vi "Auto Drive.vi"(6 "2nd Gear?":dbl, 7 "Async?":dbl, 8 "X Speed":dbl, 9 "Y Speed":dbl, 10 "Heading Target":dbl, 11 "Distance Target":dbl) -> (3 "Finished?":bool)   [LabVIEW 2017]
uses:
  Common Code/Drivetrain Mode.ctl
  Robot Global Data.vi
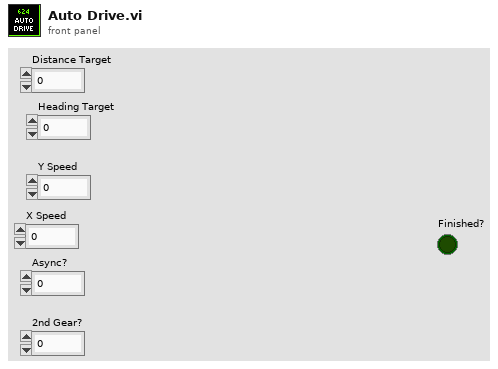
[diagram p1: front panel]
types:
  T1 = typedef "Drivetrain Mode.ctl" = enum16{"Manual", "Gyro Steer", "PID Drive", "Distance Drive", "Autonomous"}
  T2 = typedef "Dashboard Status Data.ctl" = cluster{"Elevator Status Cluster":T3, "Drivetrain Status Cluster":T6, "Intake Status Cluster":T8, "Climb Status Cluster":T11, "Intake PDP Info":T12}
  T3 = typedef "Elevator Status Cluster.ctl" = cluster{"Finished":bool, "Elevator Power":dbl, "Elevator State":T4, "Elevator Mode":T5, "Elevator Height":dbl, "At Bottom?":bool, "At Top?":bool, "Scale high?":bool, "PID Output":dbl}
  T4 = typedef "Elevator State.ctl" = enum16{"Idle", "Ground", "Mid", "Scale", "Switch"}
  T5 = typedef "Elevator Mode.ctl" = enum16{"Semi Auto", "Manual", "Auto"}
  T6 = typedef "Drivetrain Status Cluster.ctl" = cluster{"Throttle (Y)":dbl, "Steer (X)":dbl, "Drivetrain Mode":T1, "Brake?":bool, "Distance Drive Complete?":bool, "PID Drive Complete?":bool, "Creep Mode?":bool, "Gyro Steer Complete?":bool, "Gyro":dbl, "X Max Output":dbl, "X Min Output":dbl, "Y Max Output ":dbl, "Y Min Output":dbl, "Heading Target":dbl, "Distance Target":dbl, "2nd Gear":bool, "Drivetrain Encoder Values":T7}
  T7 = typedef "DT Encoder Values.ctl" = cluster{"Left Encoder":cluster{"Distance":dbl, "Speed":dbl, "Tick":dbl}, "Right Encoder":cluster{"Distance":dbl, "Speed":dbl, "Tick":dbl}}
  T8 = typedef "Intake Status Cluster.ctl" = cluster{"Intake Mode":T9, "Intake States":T10, "Intake Current Angle":dbl, "Cube In Posession?":bool, "Intake Wrist Up?":bool}
  T9 = typedef "Intake Mode.ctl" = enum16{"Auto", "Semi Auto", "Manual"}
  T10 = typedef "Intake States.ctl" = enum16{"Zero", "Override Angle", "Idle", "Drop Mid", "Drop Low", "Outtake", "Intake"}
  T11 = typedef "Climb Status Cluster.ctl" = cluster{"Climb":bool, "Time Remaining":dbl, "Button Pressed":bool}
  T12 = typedef "Intake PDP Info.ctl" = cluster{"Voltage Percent Output":dbl, "Output Voltage":dbl, "Bus Voltage":dbl, "Device ID":dbl, "Output Current":dbl, "Sensor Velocity":dbl, "Sensor Position":dbl, "Pulse Width Position":dbl, "Pulse Width Velocity":dbl, "Temperature":dbl, "Inverted?":bool}
  T13 = typedef "Drivetrain Command Cluster.ctl" = cluster{"Y Power":dbl, "Turn Power":dbl, "Drivetrain Mode":T1, "2nd Gear":bool, "Y Min Output":dbl, "Y Max Output":dbl, "X Min Output":dbl, "X Max Output":dbl, "Heading Target":dbl, "Distance Target":dbl, "Brake?":bool, "Zero Gyro":bool}
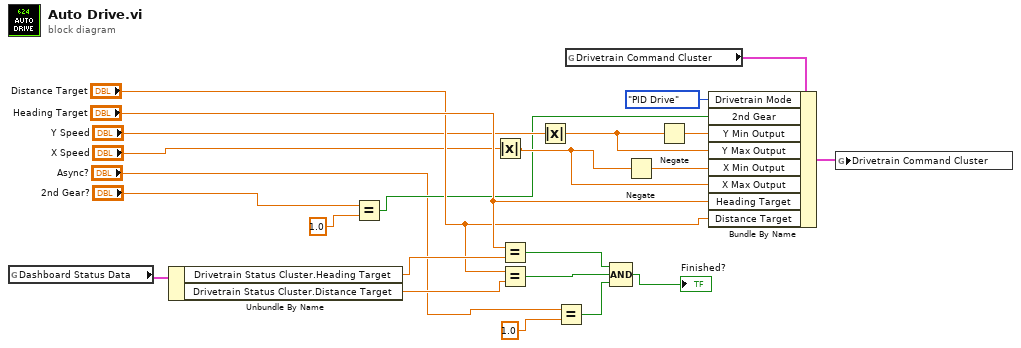
[diagram p0: block diagram]
diagram:
  n1 = global read "Robot Global Data.vi" "Dashboard Status Data"() -> (w18:T2)
  n2 = Unbundle By Name(w18) -> ("Drivetrain Status Cluster.Heading Target"=w17:dbl, "Drivetrain Status Cluster.Distance Target"=w13:dbl)
  n3 = Equal?(x="2nd Gear?", y=1.0) -> (x = y?=w5:bool)
  n4 = Absolute Value(x="X Speed") -> (abs(x)=w8:dbl)
  n5 = Equal?(x="Heading Target", y=w17) -> (x = y?=w16:bool)
  n6 = Equal?(x="Distance Target", y=w13) -> (x = y?=w12:bool)
  n7 = Absolute Value(x="Y Speed") -> (abs(x)=w10:dbl)
  n8 = Equal?(x="Async?", y=1.0) -> (x = y?=w1:bool)
  n9 = global read "Robot Global Data.vi" "Drivetrain Command Cluster"() -> (w23:T13)
  n10 = Compound Arithmetic op=AND(w16, w12, w1) -> (→"Finished?":bool)
  n11 = Negate(x=w8) -> (-x=w20:dbl)
  n12 = Negate(x=w10) -> (-x=w19:dbl)
  n13 = Bundle By Name(cluster=w23, "Drivetrain Mode"=Drivetrain_Mode."PID Drive", "2nd Gear"=w5, "Y Min Output"=w19, "Y Max Output"=w10, "X Min Output"=w20, "X Max Output"=w8, "Heading Target"="Heading Target", "Distance Target"="Distance Target") -> (w22:T13)
  n14 = global write "Robot Global Data.vi" "Drivetrain Command Cluster"(w22) -> ()
